vi "Get Thread UI.vi"(8 "error in (no error)":errorcluster, 11 "Component UI in":refnum<class "UDP User Interfaces.lvclass">) -> (0 "error out":errorcluster, 2 "Thread Settings UI":refnum<class "User Interface.lvclass">, 3 "Component UI out":refnum<class "UDP User Interfaces.lvclass">)   [LabVIEW 2020, in "UDP.lvlib" / "UDP User Interfaces.lvclass"]
uses:
  UDP User Interfaces.lvclass
  DSF Core.lvlibp/Classes/User Interface/User Interface.lvclass
  Thread/UDP Thread User Interface.lvclass
  C:/Users/nitest/Desktop/Git 2020/niveristand-data-sharing-framework-custom-device-plugins/Components/DSF Core.lvlibp/Classes/User Interface/User Interface.lvclass
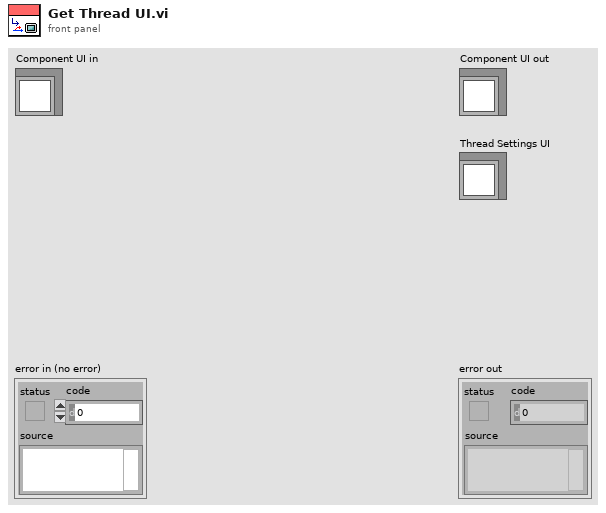
[diagram p1: front panel]
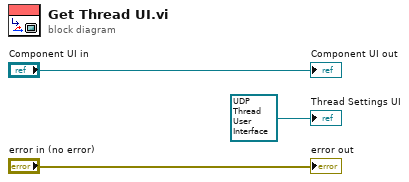
[diagram p0: block diagram]
diagram:
  "error out" <- "error in (no error)"
  "Component UI out" <- "Component UI in"
  "Thread Settings UI" <- refnum<class "UDP Thread User Interface.lvclass"> refnum ("UDP Transceiver.lvlib:UDP Thread User Interface.lvclass")
